vi "Dialog.Launch Simple Text Info Window.vi"(9 "Text":string="Info XXX", 11 "Title":string="Info") -> ()   [LabVIEW 2018]
panel:
  out "RefOut":refnum<vi>
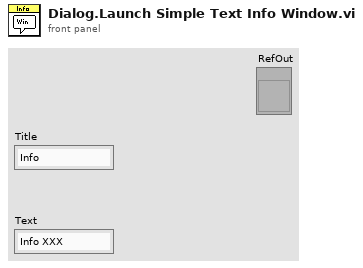
[diagram p1: front panel]
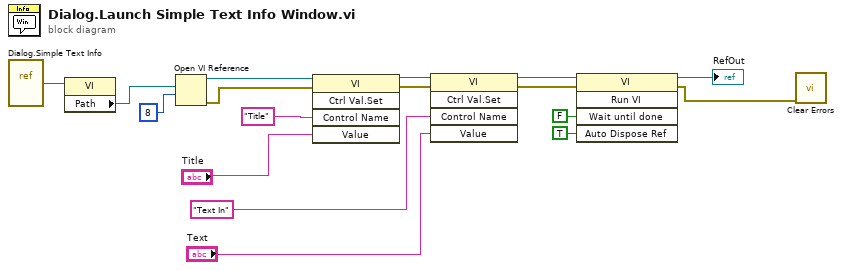
[diagram p0: block diagram]
diagram:
  n1 = vi-ref "Dialog.Simple Text Info.vi"() -> (w11:refnum<vi>)
  n2 = property class="VI"(reference=w11) -> ("Path"=w10:path)  [unwired: 1 in, 2 out]
  n3 = Open VI Reference(vi path=w10, options=8) -> (vi reference=w9:refnum<vi>, error out=w7:errorcluster)  [unwired: 4 in]
  n4 = invoke class="VI" method="Ctrl Val.Set"(reference=w9, error in=w7, "Control Name"="Title", "Value"="Title") -> (reference out=w15:refnum<vi>, error out=w14:errorcluster)  [unwired: 1 in, 3 out]
  n5 = invoke class="VI" method="Ctrl Val.Set"(reference=w15, error in=w14, "Control Name"="Text In", "Value"="Text") -> (reference out=w4:refnum<vi>, error out=w3:errorcluster)  [unwired: 1 in, 3 out]
  n6 = invoke class="VI" method="Run VI"(reference=w4, error in=w3, "Wait until done"=FALSE ("Wait Until Done"), "Auto Dispose Ref"=TRUE ("Auto Dispose Reference")) -> (reference out=→"RefOut":refnum<vi>, error out=w1:errorcluster)  [unwired: 1 in, 3 out]
  n7 = call <vilib>:"Clear Errors.vi"("error in (no error)"=w1) -> ()  [unwired: 5 in, 2 out]
